vi "Base de Datos.vi"() -> ()   [LabVIEW 2021]
uses:
  <vilib>/addons/database/Connection.llb/DB Tools Open Connec (Path).vi
  <vilib>/addons/database/Connection.llb/Conn Execute.vi
  <vilib>/addons/database/Recordset.llb/Rec Fetch String Data (R).vi
  <vilib>/addons/database/Recordset.llb/Rec Destroy - Connection.vi
  <vilib>/addons/database/NI_Database_API.lvlib
panel:
  out "String 2":string
  out "concatenated string":string
  in  "OK Button":bool
  in  "Consultar":string
  in  "Guardar Datos":bool
  out "?":bool
  in  "stop":bool
  out "Fecha y Hora":string
  in  "String":string
  in  "connection information":path
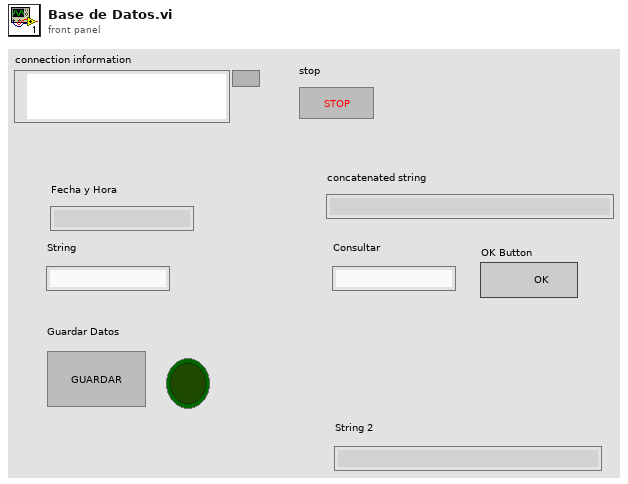
[diagram p1: front panel]
types:
  T1 = typedef "NI_Database_API.lvlib/Conn ObjectReference.ctl" = refnum<k1>
  T2 = cluster{"date/time string":string, "String":string}
  T3 = typedef "NI_Database_API.lvlib/Rec ObjectReference.ctl" = refnum<k1>
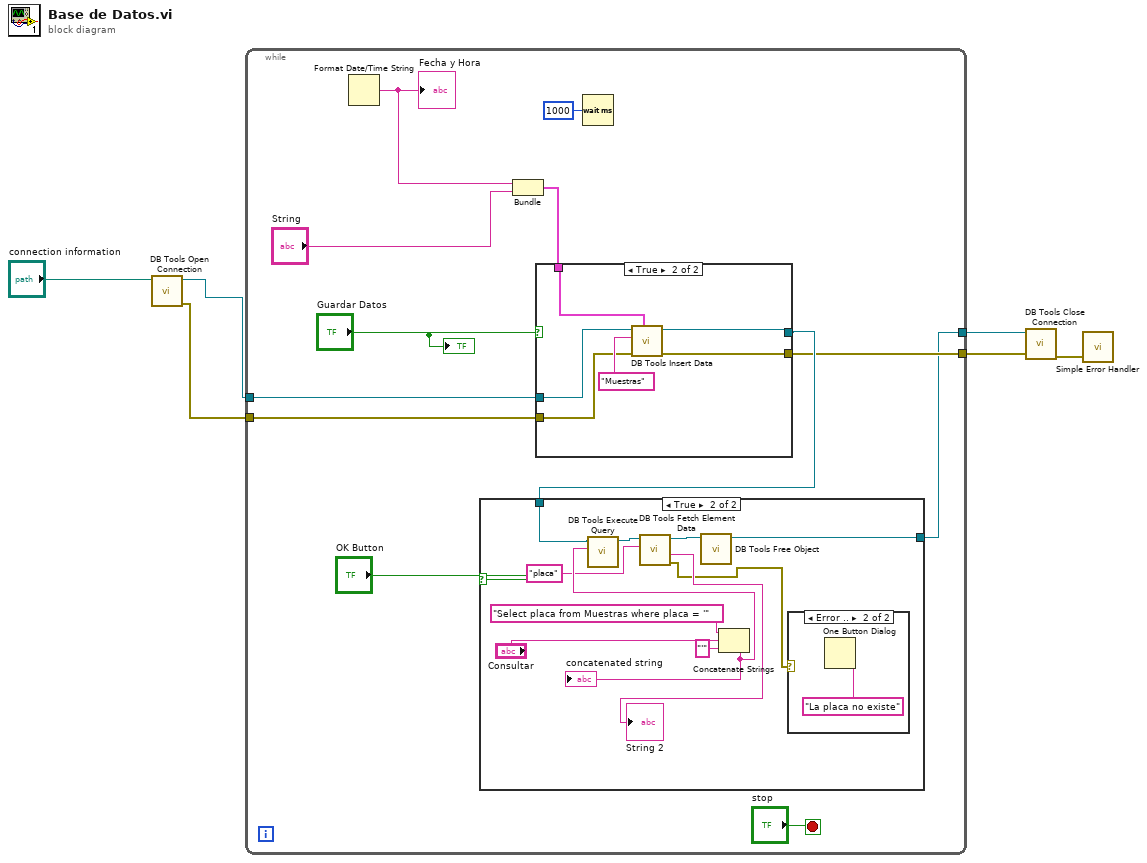
[diagram p0: block diagram]
diagram:
  n1 = call-poly <vilib>:"DB Tools Open Connection.vi"("connection information"="connection information") -> ("error out"=w3:errorcluster, "connection reference"=w5:T1)  [unwired: 7 in]
  n2 = while {
    tunnel: w5 -> [w14]
    tunnel: [w7] -> w4
    tunnel: w3 -> [w13]
    tunnel: [w8] -> w2
    stop <- "stop" stop-if-true
    n3 = Format Date/Time String() -> (date/time string=w17:string)  [unwired: 3 in]
    "Fecha y Hora" <- w17
    n4 = Bundle("date/time string"=w17, "String"="String") -> (w15:T2)  [unwired: 1 in]
    n5 = case shown="True" "Guardar Datos" {
      tunnel: w15 -> [_ w38]
      tunnel: w14 -> [w33 w39]
      tunnel: [w33 w36] -> w9
      tunnel: w13 -> [w32 w35]
      tunnel: [w32 w34] -> w8
      frame False {
      }
      frame True {
        n6 = call <vilib>:"DB Tools Insert Data.vi"("data"=w38, "error in (no error)"=w35, "table"="Muestras", "connection reference"=w39) -> ("error out"=w34:errorcluster, "connection reference out"=w36:T1)  [unwired: 6 in]
      }
    }
    n7 = case shown="True" "OK Button" {
      tunnel: w9 -> [w19 w28]
      tunnel: [w19 w26] -> w7
      frame False {
      }
      frame True {
        n8 = Concatenate Strings("Select placa from Muestras where placa = '", "Consultar", "'" ("string")) -> (w27:string)
        "concatenated string" <- w27
        n9 = call-poly <vilib>:"DB Tools Execute Query.vi"("SQL query"=w27, "connection reference"=w28) -> ("recordset reference"=w23:T3)  [unwired: 6 in, 1 out]
        n10 = call-poly <vilib>:"DB Tools Fetch Element Data.vi"("column index"="placa", "recordset reference"=w23) -> ("error out"=w20:errorcluster, "data"=→"String 2":string, "recordset reference out"=w24:T3)  [unwired: 5 in]
        n11 = call-poly <vilib>:"DB Tools Free Object.vi"("recordset reference"=w24) -> ("connection reference"=w26:T1)  [unwired: 9 in, 1 out]
        n12 = case shown="Error .." w20 {
          frame No Error {
          }
          frame Error {
            n13 = One Button Dialog(message="La placa no existe") -> ()  [unwired: 1 in, 1 out]
          }
        }
      }
    }
    n14 = Wait (ms)(milliseconds to wait=u32 1000) -> ()  [unwired: 1 out]
    "?" <- "Guardar Datos"
  }
  n15 = call <vilib>:"DB Tools Close Connection.vi"("error in (no error)"=w2, "connection reference"=w4) -> ("error out"=w1:errorcluster)  [unwired: 5 in]
  n16 = call <vilib>:"Simple Error Handler.vi"("error in (no error)"=w1) -> ()  [unwired: 4 in, 5 out]
